vi "okCFrontPanel Configure FPGA.vi"(8 "error in (no error)":errorcluster, 10 "FPGA bitfile Path":path, 11 "okCFrontPanel Device Refnum":refnum<k24>) -> (0 "error out":errorcluster, 3 "okCFrontPanel Device Refnum":refnum<k24>)   [LabVIEW 2021, in "okFrontPanelC#Wrapper.lvlib"]
uses:
  okFrontPanelC#Wrapper.lvlib
  D:/UCLA Thinkpad Google Drive/LabVIEW 2021 SP1/builds/SwissSPAD Live Distribution/Opal Kelly/C# Wrapper/v5.0.2/libFrontPanel-csharp.dll
  v5.0.2/libFrontPanel-csharp.dll
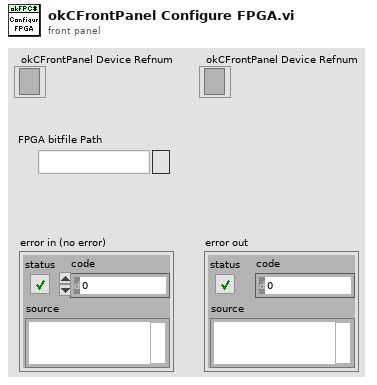
[diagram p1: front panel]
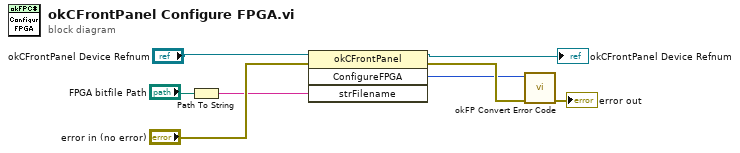
[diagram p0: block diagram]
diagram:
  n1 = Path To String(path="FPGA bitfile Path") -> (string=w4:string)
  n2 = invoke class="okCFrontPanel" method="ConfigureFPGA"(reference="okCFrontPanel Device Refnum", error in="error in (no error)", "strFilename"=w4) -> (reference out=→"okCFrontPanel Device Refnum":refnum<k24>, error out=w3:errorcluster, "ConfigureFPGA"=w2:i32)  [unwired: 1 in, 1 out]
  n3 = call "okFP Convert Error Code.vi"("error in (no error)"=w3, "okFP Error Code"=w2) -> ("error out"=→"error out":errorcluster)  [unwired: 9 in]
